vi "Message Display V1.vi"(10 "Message":string, 11 "Delay mS":dbl) -> ()   [LabVIEW 2013]
panel:
  # "USB RESET BUSY"
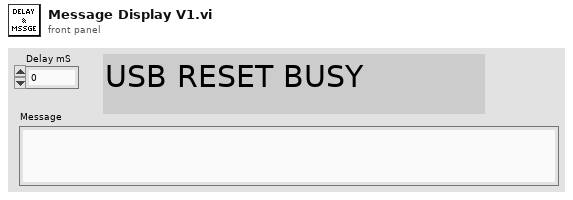
[diagram p1: front panel]
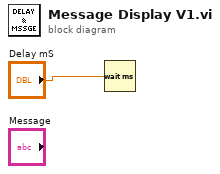
[diagram p0: block diagram]
diagram:
  n1 = Wait (ms)(milliseconds to wait="Delay mS") -> ()  [unwired: 1 out]
